vi "LuaVIEW Push (object).vi"(0 "object refnum":refnum<vi>, 1 "method table (use caller's function table)":string="caller's table", 5 "LuaVIEW reference in":T1, 11 "error in (no error)":errorcluster) -> (6 "LuaVIEW reference out":T1, 15 "error out":errorcluster)   [LabVIEW 2013]
doc: "Pushes a LuaVIEW object onto the Lua stack. To Lua it will appear as heavy userdata. This can be used to pass any refnum or other identifier specifying some LabVIEW-side object while attaching a set of methods that can be called, by Lua, on that object. The only requirement is that it can be cast into a generic refnum. Once the object is on the stack, any additional attributes can be attached using the \"Set Object Attribute\" VI. This VI is part of a polymorphic set that supports pushing various data types. To change the type being pushed, pop up on this VI's diagram icon and use the \"Select Type\" sub menu. When \"automatic\" is checked in that menu, wiring a different type to the top left input will cause the appropriate VI to be selected automatically."
uses:
  typedefs/t_LuaVIEW Reference.ctl
  typedefs/et_LuaVIEW CIN Actions.ctl
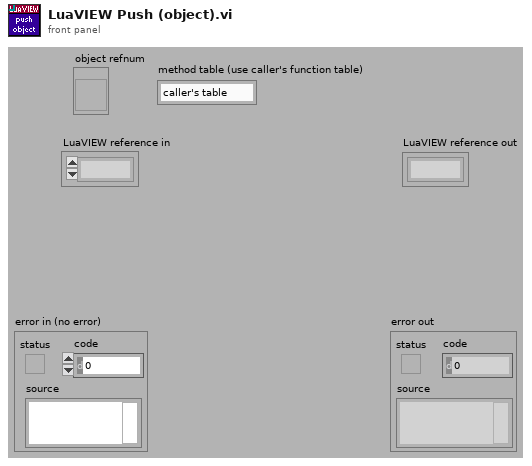
[diagram p1: front panel]
types:
  T1 = typedef "t_LuaVIEW Reference.ctl" = refnum<k1>
  T2 = typedef "et_LuaVIEW CIN Actions.ctl" = enum16{"checksynopsis", "_open", "_registerpublic", "_registerexport", "__never_an_error_result_ns", "luaversion", "cinversion", "_totals", "_taskcount", "pathological", "_unregnextpublic", "registryusecount", "__per_state_actions", "regsetprivate", "regsetindex", "regsetmodule", "_revokeexports", "_usepublic", "prepare", "compile", "execute", "call", "unregstaterefs", "_close", "pullboolean", "pullnumber", "pullI8", "pullU8", "pullI16", "pullU16", "pullI32", "pullU32", "pullobject", "pullrefnum", "pullstring", "pullflat", "pushflat", "pushobject", "getattribute", "setattribute", "stacktostring", "_startyieldtest", "_endyieldtest", "_pollprintbuffer", "__never_an_error_result_ps", "_pollexport", "setclone", "forcecleanup", "gettop", "clearstack", "insert", "pushboolean", "pushnumber", "pushrefnum", "pushstring", "pushnil", "pushvalue", "gettaskref", "settaskref"}
  T3 = typedef "et_LuaVIEW CIN Results.ctl" = enum16{"OK", "error", "main", "call", "clonecall", "modulecall", "exportcall", "index", "yield"}
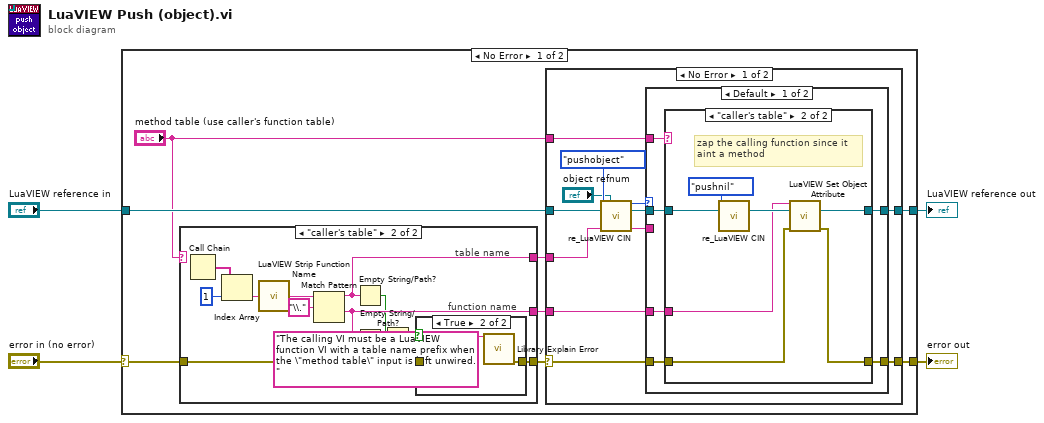
[diagram p0: block diagram]
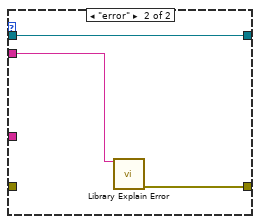
[diagram p3: hidden frame]
diagram:
  n1 = case shown="No Error" "error in (no error)" {
    selector: "error in (no error)" -> [w9 w63]
    tunnel: [w11 w62] -> w4
    tunnel: [w10 w63] -> w3
    tunnel: "LuaVIEW reference in" -> [w12 w62]
    frame No Error {
      n2 = case shown="\"caller's table\"" "method table (use caller's function table)" {
        selector: "method table (use caller's function table)" -> [w45 _]
        tunnel: w9 -> [w46 w47]
        tunnel: [w46 w53] -> w8
        tunnel: [w45 w51] -> w7
        tunnel: [_ w52] -> w5
        frame Default {
        }
        frame "caller's table" {
          # "function name"
          # "table name"
          n3 = Call Chain() -> (call chain=w58:string[])
          n4 = Index Array(array=w58, index=1) -> (element=w56:string)
          n5 = call "LuaVIEW Strip Function Name.vi"("function VI name"=w56) -> ("Lua function name"=w55:string)  [unwired: 14 in]
          n6 = Match Pattern(string=w55, regular expression="\\.") -> (before substring=w51:string, after substring=w52:string)  [unwired: 1 in, 2 out]
          n7 = Empty String/Path?(string/path=w51) -> (empty?=w50:bool)
          n8 = Empty String/Path?(string/path=w52) -> (empty?=w49:bool)
          n9 = Or(x=w50, y=w49) -> (x .or. y?=w48:bool)
          n10 = case shown="True" w48 {
            tunnel: [w59 w61] -> w53
            tunnel: w47 -> [w59 _]
            frame False {
            }
            frame True {
              n11 = call "Library Explain Error.vi"("explanation prefix (none)"="The calling VI must be a LuaVIEW function VI with a table name prefix when the \"method table\" input is left unwired." ("explanation")) -> ("explained error"=w61:errorcluster)  [unwired: 14 in]
            }
          }
        }
      }
      n12 = case shown="No Error" w8 {
        selector: w8 -> [w15 w44]
        tunnel: w12 -> [w23 w43]
        tunnel: [w19 w43] -> w11
        tunnel: [w17 w44] -> w10
        tunnel: w7 -> [w16 _]
        tunnel: "method table (use caller's function table)" -> [w14 _]
        tunnel: w5 -> [w13 _]
        frame No Error {
          n13 = call "re_LuaVIEW CIN.vi"("action"=et_LuaVIEW_CIN_Actions."pushobject", "refnum in"="object refnum", "LuaVIEW reference in"=w23, "string in"=w16) -> ("result"=w21:T3, "LuaVIEW reference out"=w20:T1, "string out"=w18:string)  [unwired: 5 in, 4 out]
          n14 = case shown="Default" w21 {
            tunnel: w20 -> [w30 w42]
            tunnel: [w29 w42] -> w19
            tunnel: w18 -> [_ w41]
            tunnel: [w25 w40] -> w17
            tunnel: w15 -> [w26 _]
            tunnel: w14 -> [w28 _]
            tunnel: w13 -> [w27 _]
            frame Default {
              n15 = case shown="\"caller's table\"" w28 {
                tunnel: w30 -> [w32 w39]
                tunnel: [w32 w35] -> w29
                tunnel: w27 -> [_ w36]
                tunnel: w26 -> [w31 w34]
                tunnel: [w31 w33] -> w25
                frame Default {
                }
                frame "caller's table" {
                  # "zap the calling function since it\naint a method"
                  n16 = call "re_LuaVIEW CIN.vi"("action"=et_LuaVIEW_CIN_Actions."pushnil", "LuaVIEW reference in"=w39) -> ("LuaVIEW reference out"=w37:T1)  [unwired: 7 in, 6 out]
                  n17 = call "LuaVIEW Set Object Attribute.vi"("key"=w36, "LuaVIEW reference in"=w37, "error in (no error)"=w34) -> ("LuaVIEW reference out"=w35:T1, "error out"=w33:errorcluster)  [unwired: 11 in]
                }
              }
            }
            frame "error" {
              n18 = call "Library Explain Error.vi"("explanation prefix (none)"=w41) -> ("explained error"=w40:errorcluster)  [unwired: 14 in]
            }
          }
        }
        frame Error {
        }
      }
    }
    frame Error {
    }
  }
  "LuaVIEW reference out" <- w4
  "error out" <- w3
